vi "Add Error.vi"(8 "error in (no error)":errorcluster, 9 "String to Append":string, 10 "Error":T1, 11 "Insert Error":bool=TRUE) -> (0 "error out":errorcluster)   [LabVIEW 2021, in "CIFCoreCommon.lvlib"]
uses:
  CIFCore/Common/CIFCoreCommon.lvlib
  Typedef/Errors.ctl
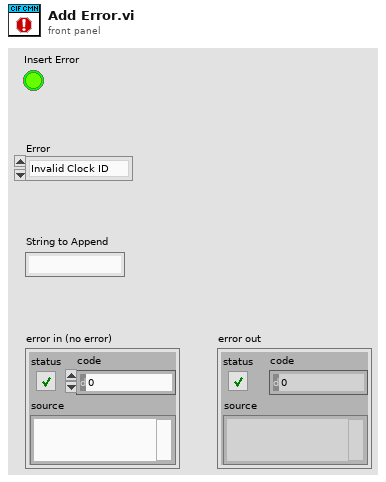
[diagram p1: front panel]
types:
  T1 = typedef "CIFCoreCommon.lvlib/Errors.ctl" = enum16{"Invalid Clock ID", "Long Sleep", "gRPC Server Not Found", "Config Parse", "Timestamp Wrap", "Delayed Execution", "Duplicate Channel", "Missing Channel", "Incorrect Type"}
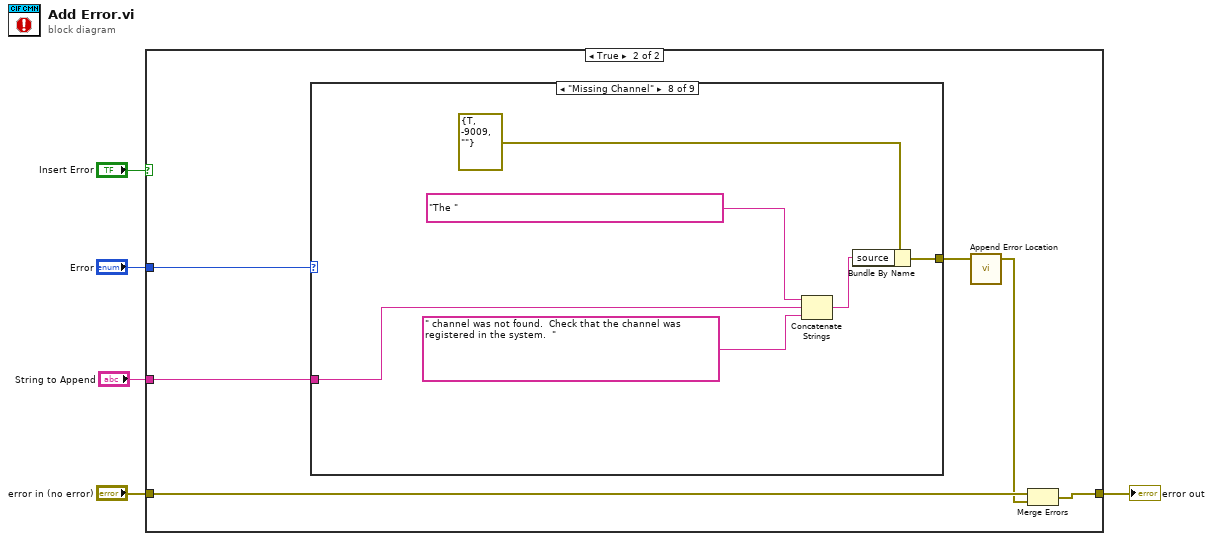
[diagram p0: block diagram]
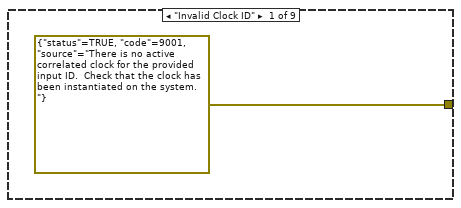
[diagram p3: hidden frame]
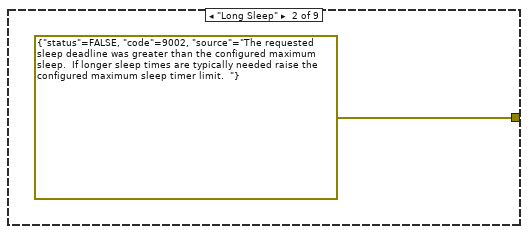
[diagram p4: hidden frame]
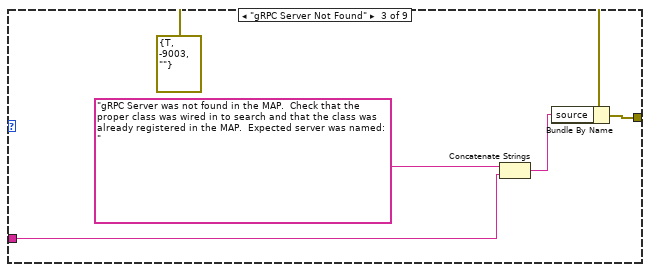
[diagram p5: hidden frame]
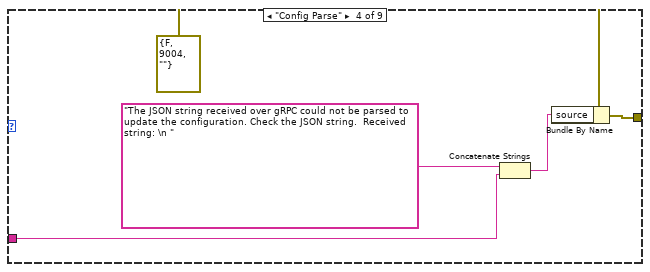
[diagram p6: hidden frame]
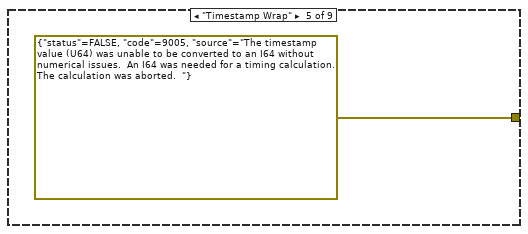
[diagram p7: hidden frame]
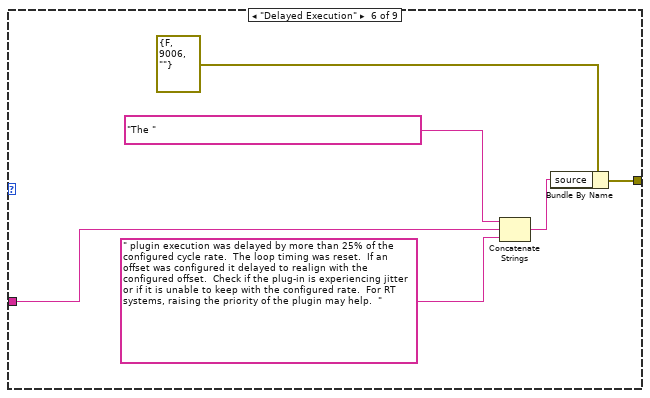
[diagram p8: hidden frame]
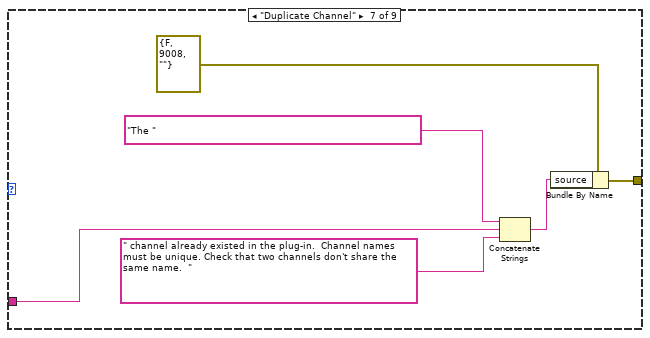
[diagram p9: hidden frame]
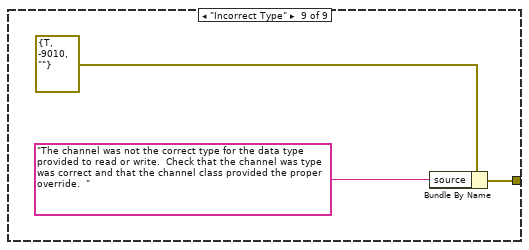
[diagram p10: hidden frame]
diagram:
  n1 = case shown="True" "Insert Error" {
    tunnel: [w6 w9] -> w4
    tunnel: "error in (no error)" -> [w6 w10]
    tunnel: "Error" -> [_ w12]
    tunnel: "String to Append" -> [_ w11]
    frame False {
    }
    frame True {
      n2 = case shown="\"Missing Channel\"" w12 {
        tunnel: w11 -> [_ _ w16 w21 _ w28 w34 w40 _]
        tunnel: [errorcluster {"status"=TRUE, "code"=9001, "source"="There is no active correlated clock for the provided input ID.  Check that the clock has been instantiated on the system.   "} ("Invalid ID") errorcluster {"status"=FALSE, "code"=9002, "source"="The requested sleep deadline was greater than the configured maximum sleep.  If longer sleep times are typically needed raise the configured maximum sleep timer limit.  "} ("Invalid ID") w18 w23 errorcluster {"status"=FALSE, "code"=9005, "source"="The timestamp value (U64) was unable to be converted to an I64 without numerical issues.  An I64 was needed for a timing calculation.  The calculation was aborted.  "} ("Invalid ID") w30 w36 w42 w45] -> w8
        frame "Invalid Clock ID" {
        }
        frame "Long Sleep" {
        }
        frame "gRPC Server Not Found" {
          n3 = Concatenate Strings("gRPC Server was not found in the MAP.  Check that the proper class was wired in to search and that the class was already registered in the MAP.  Expected server was named:  " ("source"), w16) -> (w17:string)
          n4 = Bundle By Name(cluster=errorcluster {"status"=TRUE, "code"=-9003, "source"=""} ("Invalid ID"), "source"=w17) -> (w18:errorcluster)
        }
        frame "Config Parse" {
          n5 = Concatenate Strings("The JSON string received over gRPC could not be parsed to update the configuration. Check the JSON string.  Received string: \n " ("source"), w21) -> (w22:string)
          n6 = Bundle By Name(cluster=errorcluster {"status"=FALSE, "code"=9004, "source"=""} ("Invalid ID"), "source"=w22) -> (w23:errorcluster)
        }
        frame "Timestamp Wrap" {
        }
        frame "Delayed Execution" {
          n7 = Concatenate Strings("The " ("source"), w28, " plugin execution was delayed by more than 25% of the configured cycle rate.  The loop timing was reset.  If an offset was configured it delayed to realign with the configured offset.  Check if the plug-in is experiencing jitter or if it is unable to keep with the configured rate.  For RT systems, raising the priority of the plugin may help.  " ("source")) -> (w29:string)
          n8 = Bundle By Name(cluster=errorcluster {"status"=FALSE, "code"=9006, "source"=""} ("Invalid ID"), "source"=w29) -> (w30:errorcluster)
        }
        frame "Duplicate Channel" {
          n9 = Concatenate Strings("The " ("source"), w34, " channel already existed in the plug-in.  Channel names must be unique. Check that two channels don't share the same name.  " ("source")) -> (w35:string)
          n10 = Bundle By Name(cluster=errorcluster {"status"=FALSE, "code"=9008, "source"=""} ("Invalid ID"), "source"=w35) -> (w36:errorcluster)
        }
        frame "Missing Channel" {
          n11 = Concatenate Strings("The " ("source"), w40, " channel was not found.  Check that the channel was registered in the system.  " ("source")) -> (w41:string)
          n12 = Bundle By Name(cluster=errorcluster {"status"=TRUE, "code"=-9009, "source"=""} ("Invalid ID"), "source"=w41) -> (w42:errorcluster)
        }
        frame "Incorrect Type" {
          n13 = Bundle By Name(cluster=errorcluster {"status"=TRUE, "code"=-9010, "source"=""} ("Invalid ID"), "source"="The channel was not the correct type for the data type provided to read or write.  Check that the channel was type was correct and that the channel class provided the proper override.  ") -> (w45:errorcluster)
        }
      }
      n14 = call "Append Error Location.vi"("error in (no error)"=w8) -> ("error out"=w7:errorcluster)  [unwired: 4 in]
      n15 = Merge Errors(w10, w7) -> (w9:errorcluster)
    }
  }
  "error out" <- w4
